vi "GetIniScript.vi"(8 "Error":errorcluster[](array[cluster]), 11 "Test":refnum<class "Test.lvclass">) -> (0 "Error":errorcluster[](array[cluster]), 2 "Script":string[](array[string]), 3 "Test":refnum<class "Test.lvclass">)   [LabVIEW 2014, in "Test.lvclass"]
uses:
  Test.lvclass
  Test.lvclass/Test.ctl
  Accessors/Read PluginPathArray.vi
  Accessors/Read PluginIndex.vi
  Accessors/Read ErrorSeverity.vi
  <vilib>/Utility/error.llb/Error Cluster From Error Code.vi
  <vilib>/ErrorRing/Error Ring.xnode
  <vilib>/Utility/config.llb/NI_LVConfig.lvlib
  <userlib>/NIST/NISTErrorLib/NISTErrorLib.lvlib
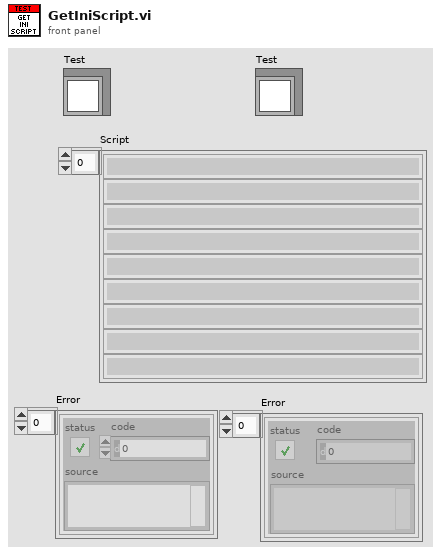
[diagram p1: front panel]
types:
  T1 = typedef "NI_LVConfig.lvlib/Config Data RefNum.ctl" = refnum<k1>
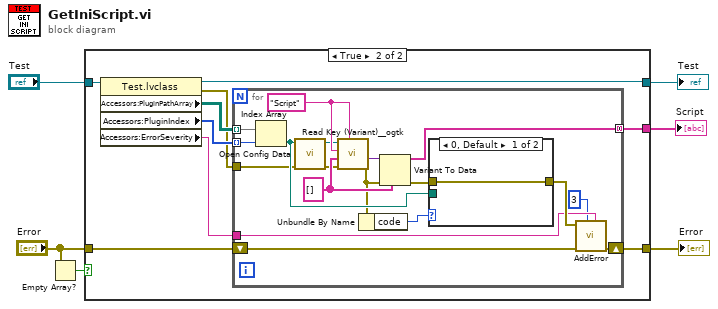
[diagram p0: block diagram]
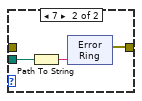
[diagram p3: hidden frame]
diagram:
  n1 = Empty Array?(array="Error") -> (empty?=w5:bool)
  n2 = case shown="True" w5 {
    tunnel: "Error" -> [w8 w13]
    tunnel: [w8 w14] -> w4
    tunnel: "Test" -> [w7 w17]
    tunnel: [w7 w11] -> w2
    tunnel: [_ w9] -> w1
    frame False {
    }
    frame True {
      n3 = property class="Test.lvclass"(reference=w17) -> (reference out=w11:refnum<class "Test.lvclass">, error out=w10:errorcluster, "Accessors:PluginPathArray"=w15:path[][], "Accessors:PluginIndex"=w16:u32[], "Accessors:ErrorSeverity"=w12:string)  [unwired: 1 in]
      n4 = for {
        tunnel: w16 -> [w35] mode=indexing
        tunnel: w15 -> [w29] mode=indexing
        shift-right: [w27] -> w14
        shift-left: w13 -> [w23]
        tunnel: w12 -> [w25]
        tunnel: [w22] -> w9 mode=concatenating
        tunnel: w10 -> [w20]
        w32 = string[] []
        w34 = "Script" ("section")
        n5 = Index Array(array=w29, index=w35) -> (element=w28:path)
        n6 = call <vilib>:"Open Config Data.vi"("error in (no error)"=w20, "configuration file path"=w28) -> ("error out"=w21:errorcluster, "refnum"=w33:T1)  [unwired: 7 in, 1 out]
        n7 = call <userlib>:"Read Key (Variant)__ogtk.vi"("section"=w34, "error in (no error)"=w21, "type"=w32, "key (optional)"=w34, "refnum"=w33) -> ("error out"=w19:errorcluster, "key-value"=w31:variant)  [unwired: 3 in, 2 out]
        n8 = Unbundle By Name(w19) -> ("code"=w18:i32)
        n9 = Variant To Data(error in=w19, type=w32, Variant=w31) -> (data=w22:string[], error out=w30:errorcluster)
        n10 = case shown="0, Default" w18 {
          tunnel: [w36 w37] -> w26
          tunnel: w28 -> [_ w38]
          tunnel: w30 -> [w36 _]
          frame 0, Default {
          }
          frame 7 {
            n11 = Path To String(path=w38) -> (string=w39:string)
            n12 = xnode "Error Ring"("parameter 0"=w39) -> ("error out"=w37:errorcluster)
          }
        }
        n13 = call <userlib>:"AddError.vi"("Severity"=w25, "Priority"=u8 3, "ErrorArray"=w23, "error in (no error)"=w26) -> ("ErrorArray"=w27:errorcluster[])  [unwired: 6 in, 1 out]
      }
    }
  }
  "Error" <- w4
  "Test" <- w2
  "Script" <- w1
